vi "ImportScan.vi"(6 "notes":string, 7 "depth":dbl, 8 "error in (no error)":errorcluster, 9 "filename":string, 10 "scan_idx":dbl, 11 "Acquisition in":refnum<class "Acquisition.lvclass">) -> (0 "error out":errorcluster, 3 "Acquisition out":refnum<class "Acquisition.lvclass">)   [LabVIEW 2014, in "Acquisition.lvclass"]
uses:
  Acquisition.lvclass
  Acquisition.lvclass/Acquisition.ctl
  Database/Database.lvclass
panel:
  in  "Tuple":T1={"mouse_id"=1217.0, "session_timestamp"="", "scan_idx"=0.0, "filename"="", "depth"=0.0, "notes"=""}
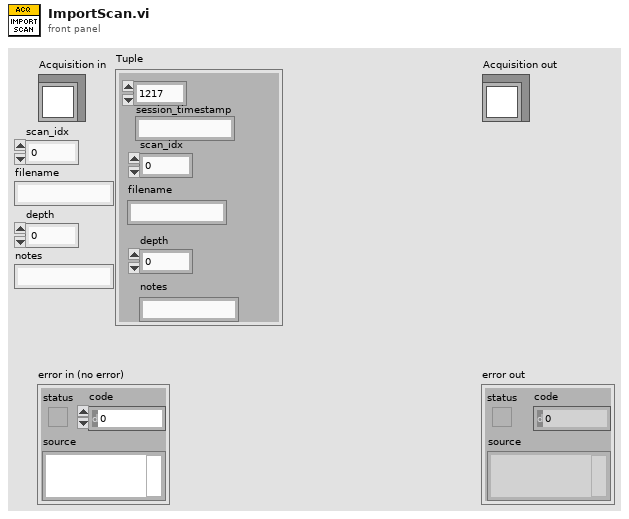
[diagram p1: front panel]
types:
  T1 = cluster{"mouse_id":dbl, "session_timestamp":string, "scan_idx":dbl, "filename":string, "depth":dbl, "notes":string}
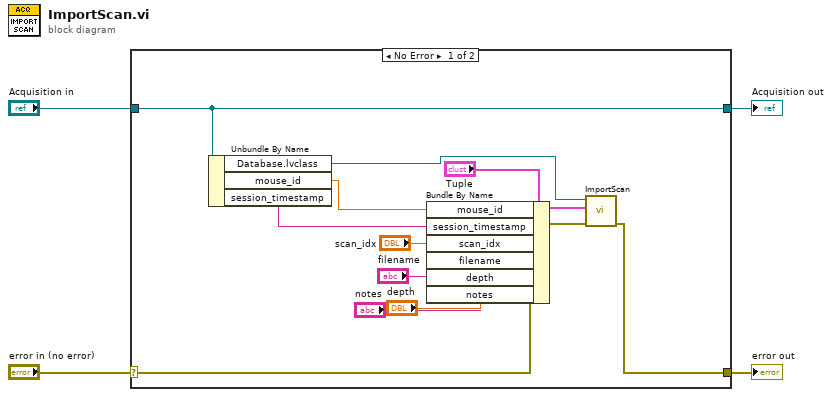
[diagram p0: block diagram]
diagram:
  n1 = case shown="No Error" "error in (no error)" {
    selector: "error in (no error)" -> [w12 w18]
    tunnel: [w11 w18] -> w3
    tunnel: [w16 w17] -> w1
    tunnel: "Acquisition in" -> [w16 w17]
    frame No Error {
      n2 = Unbundle By Name(w16) -> ("Database.lvclass"=w14:refnum<class "Database.lvclass">, "mouse_id"=w10:dbl, "session_timestamp"=w9:string)
      n3 = Bundle By Name(cluster="Tuple", "mouse_id"=w10, "session_timestamp"=w9, "scan_idx"="scan_idx", "filename"="filename", "depth"="depth", "notes"="notes") -> (w13:T1)
      n4 = call-dynamic "ImportScan.vi"("error in (no error)"=w12, "Tuple"=w13, "Database in"=w14) -> ("error out"=w11:errorcluster)  [unwired: 7 in, 1 out]
    }
    frame Error {
    }
  }
  "error out" <- w3
  "Acquisition out" <- w1
